vi "codigo 1.vi"() -> ()   [LabVIEW 2019]
panel:
  out "Numeric 2":dbl
  in  "Numeric":dbl
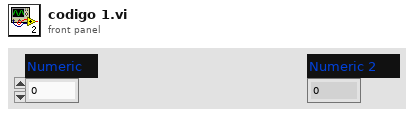
[diagram p1: front panel]
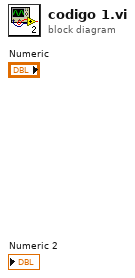
[diagram p0: block diagram]
diagram:
